vi "Get Backup.vi"(8 "error in (no error)":errorcluster, 9 "to":timestamp format="%<%x>T", 10 "from":timestamp format="%<%x>T", 11 "eLab in":refnum<class "PL eLabFTW Client.lvclass">) -> (0 "error out":errorcluster, 2 "data":string, 3 "eLab out":refnum<class "PL eLabFTW Client.lvclass">)   [LabVIEW 2015, in "PL eLabFTW Client.lvclass"]
doc: "Saves backup with the experiments for the specified time period to the specified path. The backup is ordered by users and contains only the experiments that changed in the specified time period."
uses:
  PL eLabFTW Client.lvclass
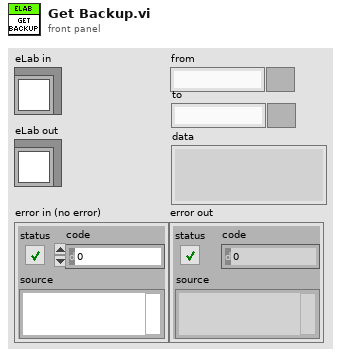
[diagram p1: front panel]
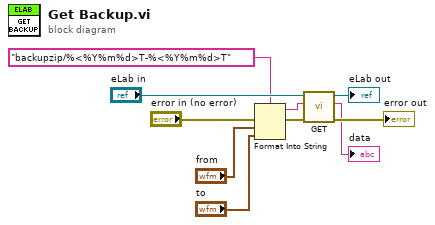
[diagram p0: block diagram]
diagram:
  n1 = Format Into String(format string="backupzip/%<%Y%m%d>T-%<%Y%m%d>T", error in="error in (no error)", "from", "to") -> (resulting string=w8:string, error out=w7:errorcluster)  [unwired: 1 in]
  n2 = call "GET.vi"("error in (no error)"=w7, "relative URL"=w8, "eLab in"="eLab in") -> ("error out"=→"error out":errorcluster, "response body"=→"data":string, "eLab out"=→"eLab out":refnum<class "PL eLabFTW Client.lvclass">)  [unwired: 6 in]
